vi "BadAiMax Filter.vi"(8 "error in (no error)":errorcluster, 9 "Max In":dbl, 10 "Min In":dbl, 11 "Channel Name":string) -> (0 "error out":errorcluster, 1 "Max Out":dbl, 2 "Min Out":dbl)   [LabVIEW 2013]
uses:
  Data Access Objects/Sensors/Sensor DB Actions.ctl
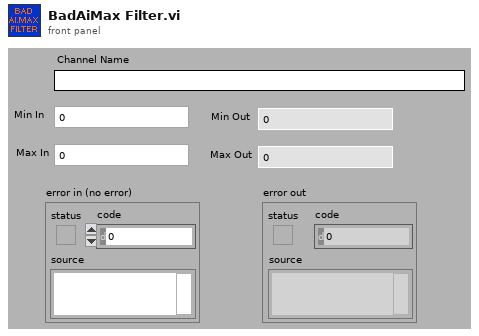
[diagram p1: front panel]
types:
  T1 = typedef "Sensor DB Actions.ctl" = enum16{"Init", "Set ", "Get ", "Save", "Load", "Remove"}
  T2 = typedef "Sensor Limit.ctl" = cluster{"Upper":dbl, "Lower":dbl}
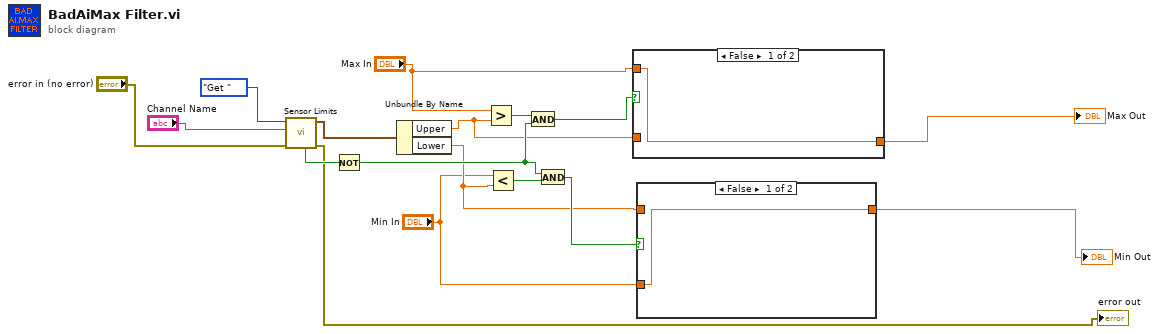
[diagram p0: block diagram]
diagram:
  n1 = call "Sensor Limits.vi"("error in (no error)"="error in (no error)", "Channel Path"="Channel Name", "Sensor Actions"=Sensor_DB_Actions."Get ") -> ("error out"=→"error out":errorcluster, "Limits Out"=w14:T2, "Not Found"=w11:bool)  [unwired: 5 in, 1 out]
  n2 = Not(x=w11) -> (.not. x?=w10:bool)
  n3 = Unbundle By Name(w14) -> ("Upper"=w7:dbl, "Lower"=w2:dbl)
  n4 = Greater?(x="Max In", y=w7) -> (0:w13:bool)
  n5 = Less?(x="Min In", y=w2) -> (x < y?=w12:bool)
  n6 = And(x=w13, y=w10) -> (x .and. y?=w9:bool)
  n7 = And(x=w10, y=w12) -> (x .and. y?=w8:bool)
  n8 = case shown="False" w9 {
    tunnel: w7 -> [_ w19]
    tunnel: "Max In" -> [w18 _]
    tunnel: [w18 w19] -> w5
    frame False {
    }
    frame True {
    }
  }
  "Max Out" <- w5
  n9 = case shown="False" w8 {
    tunnel: "Min In" -> [w20 _]
    tunnel: w2 -> [_ w21]
    tunnel: [w20 w21] -> w4
    frame False {
    }
    frame True {
    }
  }
  "Min Out" <- w4
